vi "DI Interrupt Handling.vi"() -> ()   [LabVIEW 2021]
uses:
  <vilib>/myRIO/Instrument Drivers/Utilities/Utilities.lvlib
  <vilib>/Platform/TimedLoop/XDataNode/wakeup.ctl
  <vilib>/Platform/TimedLoop/XDataNode/XDNodeRunTimeDep.lvlib
  <vilib>/Platform/TimedLoop/XDataNode/nitl_modes.ctl
  <vilib>/Platform/TimedLoop/XDataNode/timing_clust.ctl
  <vilib>/Platform/TimedLoop/XDataNode/XDataNode.xnode
  <vilib>/myRIO/Express VI/IRQ/IRQ Express VI.xnode
  <vilib>/myRIO/Common/Instrument Driver Framework/myRIO v1.0/IRQ/typedefs/DI IRQ Type.ctl
  <vilib>/myRIO/Common/Instrument Driver Framework/myRIO v1.0/IRQ/typedefs/Callback VI Ref.ctl
  <vilib>/myRIO/Instrument Drivers/IRQ/IO IRQ/vis/myRIO Register DI IRQ.xnode
  <vilib>/myRIO/Common/Instrument Driver Framework/myRIO v1.0/IRQ/vis/myRIO v1.1 Register DI IRQ.vi
  <vilib>/userdefined/High Color/nirio_resource_hc.ctl
  DI Callback 1 CPU.vi
  DI Callback 2 CPUs.vi
  <vilib>/myRIO/Express VI/Onboard IO/DI/DI Express VI.xnode
  <vilib>/myRIO/Instrument Drivers/Onboard IO/DIO/vis/Read.vi
  <vilib>/myRIO/Instrument Drivers/Onboard IO/DIO/DIO.lvlib
  <vilib>/myRIO/Common/Instrument Driver Framework/myRIO v1.0/DIO/typedefs/DIO Channels Enum.ctl
  <vilib>/myRIO/Common/Instrument Driver Framework/myRIO v1.0/DIO/typedefs/DIO Channels List.ctl
  <vilib>/myRIO/Common/Instrument Driver Framework/Utilities/typedefs/Generic FPGA Reference.ctl
  <vilib>/myRIO/Common/Instrument Driver Framework/Utilities/typedefs/myRIO v1.0 Reference.ctl
  <vilib>/myRIO/Common/Instrument Driver Framework/Utilities/typedefs/Hardware Version Enum.ctl
  <vilib>/myRIO/Common/Instrument Driver Framework/Utilities/typedefs/myRIO Generic Hardware Reference.ctl
  <vilib>/myRIO/Instrument Drivers/Onboard IO/DIO/typedefs/DIO Reference.ctl
  <vilib>/myRIO/Instrument Drivers/Onboard IO/DIO/vis/myRIO DIO Open.xnode
  <vilib>/myRIO/Common/Instrument Driver Framework/Utilities/vis/Is FPGA Ref Available.vi
  <vilib>/myRIO/Common/Instrument Driver Framework/myRIO v1.0/DIO/vis/myRIO v1.1 Open DIO.vi
panel:
  in  "Mode":T1(ring)
  out "Waveform Chart":cluster{i16, "element":i16}(graph)
  in  "stop":bool
  out "error out":errorcluster
  # "Overview: This VI demonstrates how to use callback VIs to handle a digital input interrupt.\nInstructions:\n1.\tConnect an external digital signal to the A/DIO0 (Pin 11) with a cable. A/ stands for connector A on the myRIO.\n2.\tIn the Project Explorer window, verify the IP address of the myRIO target. If it is incorrect, update the IP address.\n3.\tRun the VI.\n4.\tThe waveform displays the digital input signal that the VI reads on the DIO0 channel.\n5.\tThe edge count for triggering the digital input is two. The VI triggers an interrupt on the rising edge of the digital input signal. Thus, every time when the digital input signal meets both prerequisites, an impulse appears on the trigger point in the waveform chart.\n6.\tThe VI includes two callback VIs. One VI uses one CPU, whereas the other VI uses two CPUs. To see the different impacts between the two modes, change the value of Mode."
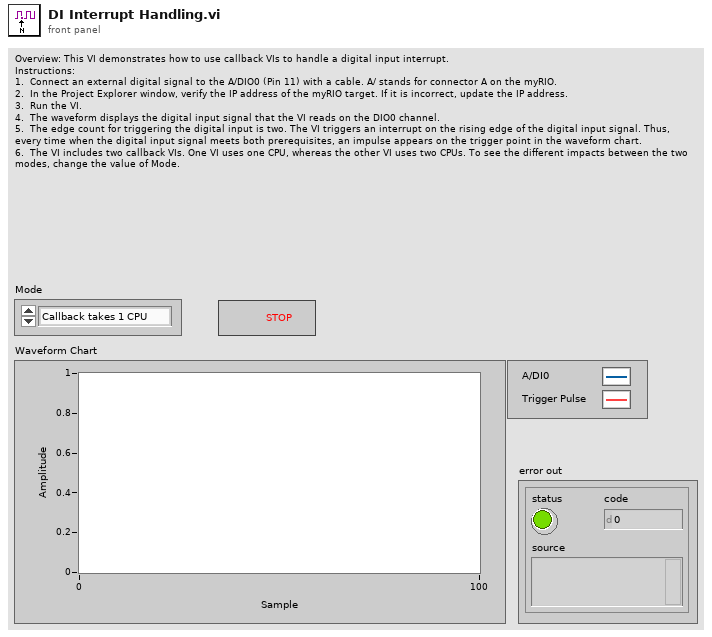
[diagram p1: front panel]
types:
  T1 = enum16{"Callback takes 1 CPU", "Callback takes 2 CPUs"}
  T2 = typedef "DI IRQ Type.ctl" = enum16{"Digital falling edge", "Digital rising edge", "Digital edge"}
  T3 = typedef "nirio_resource_hc.ctl" = tag
  T4 = typedef "DIO.lvlib/DIO Reference.ctl" = cluster{"myRIO Reference":T5, "DIO Channels List":T9}
  T5 = typedef "myRIO Generic Hardware Reference.ctl" = cluster{"myRIO Model":T6, "myRIO Hardware Reference":T7}
  T6 = typedef "Hardware Version Enum.ctl" = enum16{"Unknown", "myRIO-1900", "myRIO-1950", "roboRIO", "NI ELVIS RIO CM", "ELVIS III"}
  T7 = typedef "myRIO v1.0 Reference.ctl" = cluster{"Generic FPGA Reference":T8, "Allow multiple opens":bool}
  T8 = typedef "Generic FPGA Reference.ctl" = refnum<k20>
  T9 = typedef "DIO Channels List.ctl" = T10[]
  T10 = typedef "DIO Channels Enum.ctl" = enum16{"Not Connected", "C/DIO0", "C/DIO1", "C/DIO2", "C/DIO3", "C/DIO4", "C/DIO5", "C/DIO6", "C/DIO7", "A/DIO0", "A/DIO1", "A/DIO2", "A/DIO3", "A/DIO4", "A/DIO5", "A/DIO6", "A/DIO7", "A/DIO8", "A/DIO9", "A/DIO10", "A/DIO11", "A/DIO12", "A/DIO13", "A/DIO14", "A/DIO15", "A/DIO16", "A/DIO17", "A/DIO18", "A/DIO19", "B/DIO0", "B/DIO1", "B/DIO2", "B/DIO3", "B/DIO4", "B/DIO5", "B/DIO6", "B/DIO7", "B/DIO8", "B/DIO9", "B/DIO10", "B/DIO11", "B/DIO12", "B/DIO13", "B/DIO14", "B/DIO15", "B/DIO16", "B/DIO17", "B/DIO18", "B/DIO19", "LED0", "LED1", "LED2", "LED3", "Button0", "DIO/DIO0", "DIO/DIO1", "DIO/DIO2", "DIO/DIO3", "DIO/DIO4", "DIO/DIO5", "DIO/DIO6", "DIO/DIO7", "DIO/DIO8", "DIO/DIO9", "SPI/CS0", "SPI/CS1", "SPI/CS2", "SPI/CS3", "LED RADIO (Green)", "LED RADIO (Red)", "LED COMM (Green)", "LED COMM (Red)", "LED MODE (Green)", "LED MODE (Red)"}
  T11 = typedef "XDNodeRunTimeDep.lvlib/timing_clust.ctl" = cluster{"Expected End [f-1]":u64, "Actual End [f-1]":u64, "Finished Late? [f-1]":bool, "Expected End [i-1]":u64, "Actual End [i-1]":u64, "Finished Late? [i-1]":bool, "Expected Start [i]":u64, "Actual Start [i]":u64, "Expected Start [f]":u64, "Actual Start [f]":u64, "Source Name":string, "Structure Name":string, "Period":i64, "Deadline":i64, "Offset":i64, "Start":i64, "Priority":i32, "Timeout":i32, "Mode":T12, "Wakeup Reason":T13, "Error":errorcluster, "Source Type":string, "Secondary Source Type":string, "Global End Time":u64, "Global Start Time":u64, "Frame Duration":u64, "Iteration Duration":u64, "Assigned CPU":i32, "I/O Scan Engine Mode":u32}
  T12 = typedef "XDNodeRunTimeDep.lvlib/nitl_modes.ctl" = enum32{"No Change", "Process missed periods, maintain original phase", "Discard missed periods, maintain original phase", "Process missed periods, ignore original phase", "Discard missed periods, ignore original phase"}
  T13 = typedef "XDNodeRunTimeDep.lvlib/wakeup.ctl" = enum32{"Normal", "Aborted", "Asynchronous wakeup", "Timing source error", "Timed loop error", "Timeout"}
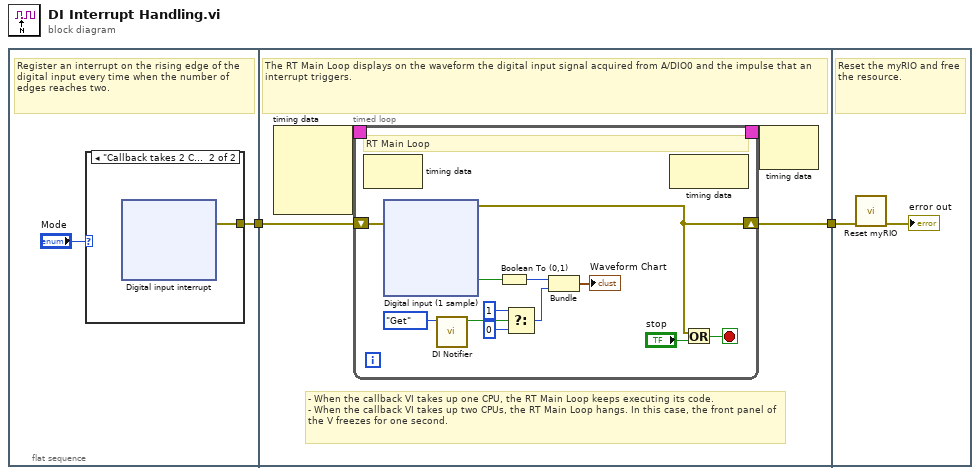
[diagram p0: block diagram]
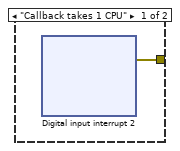
[diagram p2: hidden frame]
diagram:
  n1 = flat-sequence {
    tunnel: [w4] -> w2
    tunnel: w2 -> [w42]
    tunnel: [w41] -> w1
    tunnel: w1 -> [w96]
    frame #0 {
      # "Register an interrupt on the rising edge of the digital input every time when the number of edges reaches two."
      n2 = case shown="\"Callback takes 2 CPUs\"" "Mode" {
        tunnel: [w5 w23] -> w4
        frame "Callback takes 1 CPU" {
          n3 = xnode "Digital input interrupt 2"() -> ("error out"=w5:errorcluster)  [unwired: 1 in]
        }
        frame "Callback takes 2 CPUs" {
          n4 = xnode "Digital input interrupt"() -> ("error out"=w23:errorcluster)  [unwired: 1 in]
        }
      }
    }
    frame #1 {
      # "- When the callback VI takes up one CPU, the RT Main Loop keeps executing its code.\n- When the callback VI takes up two CPUs, the RT Main Loop hangs. In this case, the front panel of the V freezes for one second."
      # "The RT Main Loop displays on the waveform the digital input signal acquired from A/DIO0 and the impulse that an interrupt triggers."
      n5 = node-c288() -> (w44:T11)  [unwired: 4 in]
      n6 = timed-loop {
        timing: w44 -> [_]
        timing-out: [_] -> w43
        shift-right: [w46] -> w41
        shift-left: w42 -> [w47]
        stop <- w55 stop-if-true
        # "RT Main Loop"
        n7 = node-c288() -> ()  [unwired: 1 in, 1 out]
        n8 = xnode "Digital input (1 sample)"("error in (no error)"=w47) -> ("A/DIO0 (Pin 11)"=w45:bool, "error out"=w46:errorcluster)
        n9 = call "DI Notifier.vi"("Action"=enum16{"Get", "Set"}."Get") -> ("Trigger?"=w51:bool)  [unwired: 10 in]
        n10 = Boolean To (0,1)(Boolean=w45) -> (0, 1=w50:i16)
        n11 = Select(t=i16 1 ("element"), s=w51, f=i16 0 ("element")) -> (s? t:f=w49:i16)
        n12 = Bundle(w50, "element"=w49) -> (→"Waveform Chart":cluster{i16, "element":i16})  [unwired: 1 in]
        n13 = node-c288() -> ()  [unwired: 1 in, 1 out]
        n14 = Or(x=w46, y="stop") -> (x .or. y?=w55:bool)
      }
      n15 = node-c288(w43) -> ()  [unwired: 1 out]
    }
    frame #2 {
      # "Reset the myRIO and free the resource."
      n16 = call <vilib>:"Reset myRIO.vi"("error in (no error)"=w96) -> ("error out"=→"error out":errorcluster)  [unwired: 10 in]
    }
  }
